vi "Caller.vi"   [LabVIEW 2017]
uses:
  <userlib>/_NEVSTOP/Communicable State Machine(CSM)/Communicable State Machine.lvlib
  INI-Static-Variable-Support/INI-Static-Variable-Support.lvlib
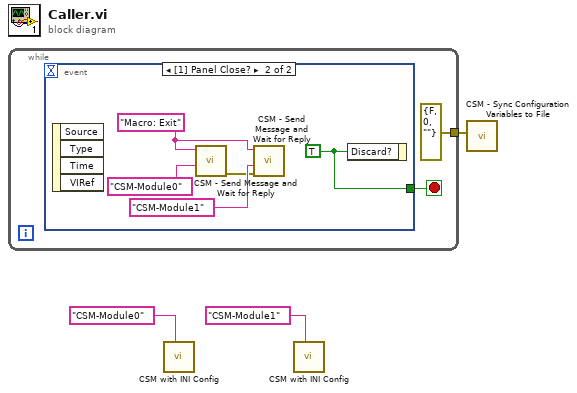
[diagram p0: block diagram]
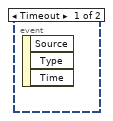
[diagram p2: hidden frame]
diagram:
  n1 = while {
    tunnel: [errorcluster {"status"=FALSE, "code"=0, "source"=""} ("error in (no error)")] -> w1
    stop <- w5 stop-if-true
    n2 = event shown="[1] Panel Close?" {
      selector: _ -> [_ _]
      dyn-events: _ -> [_ _]
      timeout: _ -> [_ _]
      tunnel: [_ w10] -> w5
      event Timeout {
        n3 = event-data() -> ()  [unwired: 1 in, 3 out]
      }
      event Panel Close? {
        w8 = "Macro: Exit" ("Arguments (\"\")")
        w10 = TRUE ("Discard?")
        n4 = event-data() -> ()  [unwired: 1 in, 4 out]
        n5 = call <userlib>:"CSM - Send Message and Wait for Reply.vi"("Target Module"="CSM-Module0" ("Name(\"\" to use uuid)"), "State"=w8) -> ("error out"=w6:errorcluster)  [unwired: 7 in, 2 out]
        n6 = call <userlib>:"CSM - Send Message and Wait for Reply.vi"("Error In (no error)"=w6, "Target Module"="CSM-Module1" ("Name(\"\" to use uuid)"), "State"=w8) -> ()  [unwired: 6 in, 3 out]
        n7 = event-data("Discard?"=w10) -> ()  [unwired: 1 in, 1 out]
      }
    }
  }
  n8 = call "CSM with INI Config.vi"("Name(\"\" to use uuid)"="CSM-Module0" ("Name(\"\" to use uuid)")) -> ()  [unwired: 11 in]
  n9 = call "CSM with INI Config.vi"("Name(\"\" to use uuid)"="CSM-Module1" ("Name(\"\" to use uuid)")) -> ()  [unwired: 11 in]
  n10 = call "CSM - Sync Configuration Variables to File.vi"("error in (no error)"=w1) -> ()  [unwired: 8 in, 1 out]
